vi "Configure Modules from Switches JSON.vi"() -> ()   [LabVIEW 2017]
uses:
  SubVIs/SLSC Switch Offline Configuration Information.ctl
  NationalInstruments.VeriStand.SystemDefinitionAPI
  <vilib>/addons/VeriStand Custom Device Scripting APIs/SLSC Switch/Shared/VeriStand SLSC Scripting/VeriStand SLSC Scripting.lvlib
  <vilib>/addons/VeriStand Custom Device Scripting APIs/SLSC Switch/SLSC Switch/Scripting/SLSC Switch Scripting.lvlib
  SLSC Switch Examples.lvlib
panel:
  in  "SLSC Chassis Name or IP":string
  in  "Controller Name":string
  in  "Custom Device Configuration":T1[](array[typedef])
  in  "Output System Definition file":path
  in  "Input System Definition File":path
  # "Overview: Demonstrates using the SLSC Switch custom device scripting API to configure instances of the custom device without requiring the hardware be present. By default, the configuration is for an NI SLSC-12251.\n\nInstructions:\n1. Browse to the system definition file to be used as input.\n2. Browse to a path to save the system definition file as output. This may be the same as the input file.\n3. Set the name of the controller in the system definition file that contains the SLSC Chassis\nand the SLSC Chassis identifier used in the system definition file. \n4. Select the slot number, model number, and resource/device name to script into the system definition file. \n5. Browse to the JSON file containing the switch definition, typically provided by the vendor.\n6. Repeat steps 4. and 5. for each custom device you wish to configure\n7. Run the VI and verify its results."
  # "System Definition Files"
  # "SLSC Chassis"
  # "Custom Device Configuration"
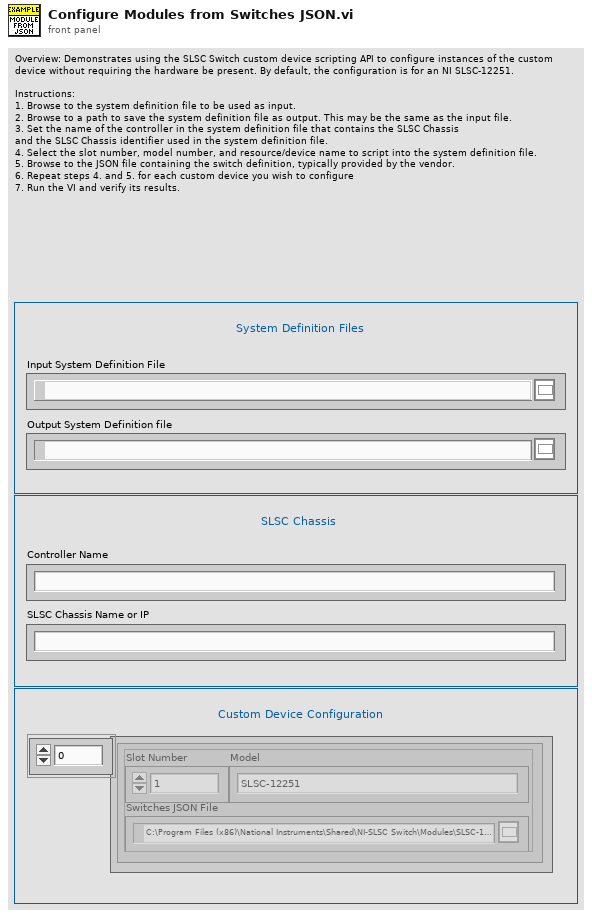
[diagram p1: front panel]
types:
  T1 = typedef "SLSC Switch Examples.lvlib/SLSC Switch Offline Configuration Information.ctl" = cluster{"Switches JSON File":path, "Slot Number":u32, "Model":string}
  T2 = typedef "Custom Device API.lvlib/Custom Device Item Ref.ctl" = u64
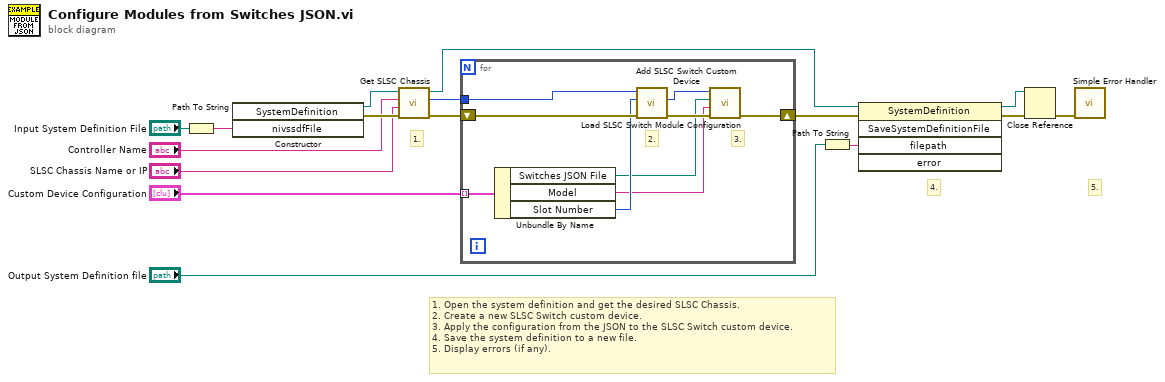
[diagram p0: block diagram]
diagram:
  # "1."
  # "4."
  # "5."
  # "1. Open the system definition and get the desired SLSC Chassis.\n2. Create a new SLSC Switch custom device.\n3. Apply the configuration from the JSON to the SLSC Switch custom device.\n4. Save the system definition to a new file.\n5. Display errors (if any)."
  n1 = Path To String(path="Input System Definition File") -> (string=w9:string)
  n2 = constructor class="SystemDefinition"("nivssdfFile"=w9) -> (reference out=w7:refnum<k24>, error out=w8:errorcluster)  [unwired: 3 in, 2 out]
  n3 = call <vilib>:"Get SLSC Chassis.vi"("error in (no error)"=w8, "SLSC Chassis Name or IP"="SLSC Chassis Name or IP", "Target Name"="Controller Name", "SysDef in"=w7) -> ("error out"=w3:errorcluster, "SLSC Chassis"=w2:u64, "SysDef out"=w1:refnum<k24>)  [unwired: 4 in, 1 out]
  n4 = for {
    shift-right: [w21] -> w12
    shift-left: w3 -> [w23]
    tunnel: "Custom Device Configuration" -> [w25] mode=indexing
    tunnel: w2 -> [w24]
    # "3."
    # "2."
    n5 = Unbundle By Name(w25) -> ("Switches JSON File"=w18:path, "Model"=w17:string, "Slot Number"=w19:u32)
    n6 = call <vilib>:"Add SLSC Switch Custom Device.vi"("error in (no error)"=w23, "Slot Number"=w19, "SLSC Chassis Ref"=w24) -> ("error out"=w22:errorcluster, "SLSC Switch Custom Device Ref"=w20:T2)  [unwired: 6 in, 1 out]
    n7 = call <vilib>:"Load SLSC Switch Module Configuration.vi"("error in"=w22, "Model"=w17, "switches JSON file"=w18, "SLSC Switch Custom Device Ref in"=w20) -> ("error out"=w21:errorcluster)  [unwired: 6 in, 1 out]
  }
  n8 = Path To String(path="Output System Definition file") -> (string=w16:string)
  n9 = invoke class="SystemDefinition" method="SaveSystemDefinitionFile"(reference=w1, error in=w12, "filepath"=w16) -> (reference out=w14:refnum<k24>, error out=w15:errorcluster)  [unwired: 2 in, 3 out]
  n10 = Close Reference(reference=w14, error in (no error)=w15) -> (error out=w11:errorcluster)
  n11 = call <vilib>:"Simple Error Handler.vi"("error in (no error)"=w11) -> ()  [unwired: 1 in, 8 out]
